vi "Initialize.vi"(8 "error in (no error)":errorcluster, 10 "Port (81)":u16=81, 11 "WebSocket In":refnum<class "Websocket.lvclass">) -> (0 "error out":errorcluster, 3 "WebSocket Out":refnum<class "Websocket.lvclass">)   [LabVIEW 2015, in "Front Panel Publisher.lvlib" / "Websocket.lvclass"]
uses:
  Websocket.lvclass
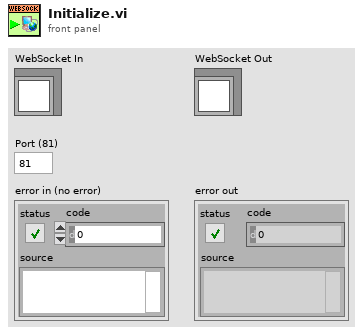
[diagram p1: front panel]
types:
  T1 = typedef "FrontPanelPublisher.lvlib/Websocket.lvclass/ObjectAttributes.ctl" = cluster{"Port":u16, "TCP Refs":refnum<k5>[], "Connection IDs":u64[]}
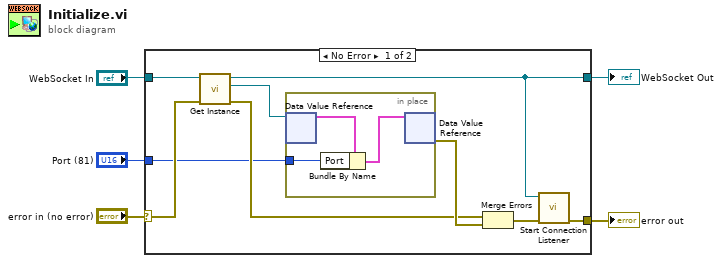
[diagram p0: block diagram]
diagram:
  n1 = case shown="No Error" "error in (no error)" {
    selector: "error in (no error)" -> [w11 w19]
    tunnel: [w6 w19] -> w4
    tunnel: "WebSocket In" -> [w10 w18]
    tunnel: [w7 w18] -> w2
    tunnel: "Port (81)" -> [w8 _]
    frame No Error {
      n2 = call "Get Instance.vi"("error in (no error)"=w11, "WebSocket In"=w10) -> ("error out"=w13:errorcluster, "DVRRefOut"=w9:refnum<data-value>, "WebSocket Out"=w7:refnum<class "Websocket.lvclass">)  [unwired: 5 in, 2 out]
      n3 = in-place {
        in-place-border: w8 -> [w15]
        n4 = in-place-dvr #1(w9) -> (w16:T1)  [unwired: 1 out]
        n5 = Bundle By Name(cluster=w16, "Port"=w15) -> (w17:T1)
        n6 = in-place-dvr #1(w17) -> (w14:errorcluster)  [unwired: 1 out]
      }
      n7 = Merge Errors(w13, w14) -> (w12:errorcluster)
      n8 = call "Start Connection Listener.vi"("error in (no error)"=w12, "Websocket In"=w7) -> ("error out"=w6:errorcluster)  [unwired: 7 in, 2 out]
    }
    frame Error {
    }
  }
  "error out" <- w4
  "WebSocket Out" <- w2
